vi "Listbox.vi"(0 "Items":i32(listbox), 5 "Selected Item":string, 7 "error in (no error)":errorcluster) -> (4 "error out":errorcluster)   [LabVIEW 2020]
doc: "This VI has a string control which moves over the row selected in the listbox."
panel:
  # "Select a row to get the string control \nover the selected row."
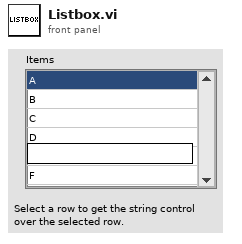
[diagram p1: front panel]
types:
  T1 = typedef "LVPositionTypeDef.ctl" = cluster{"Left":i32, "Top":i32}
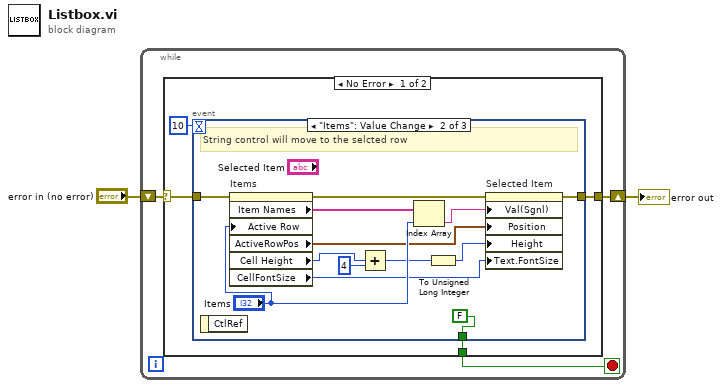
[diagram p0: block diagram]
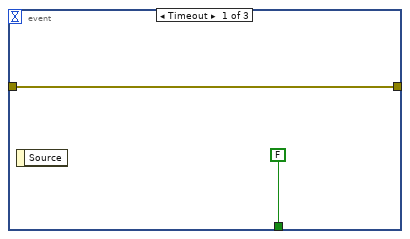
[diagram p2: hidden frame]
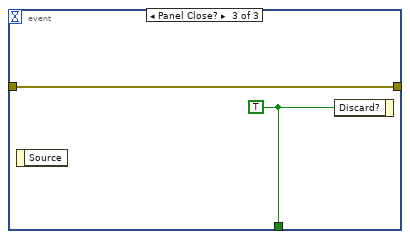
[diagram p3: hidden frame]
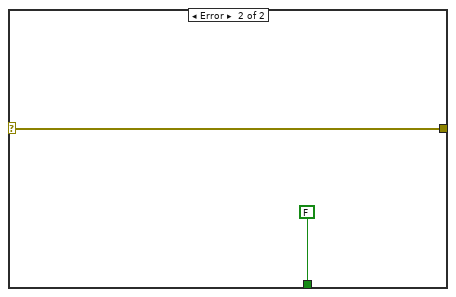
[diagram p4: hidden frame]
diagram:
  n1 = while {
    shift-right: [w5] -> w2
    shift-left: "error in (no error)" -> [w4]
    stop <- w3 stop-if-true
    n2 = case shown="No Error" w4 {
      selector: w4 -> [w8 w28]
      tunnel: [w9 w28] -> w5
      tunnel: [w6 FALSE ("Discard?")] -> w3
      frame No Error {
        n3 = event shown="[1] \"Items\": Value Change" {
          selector: _ -> [_ _ _]
          dyn-events: _ -> [_ _ _]
          timeout: 10 -> [_ _ _]
          tunnel: w8 -> [w11 w22 w25]
          tunnel: [w11 w21 w25] -> w9
          tunnel: [FALSE ("Discard?") FALSE ("Discard?") w26] -> w6
          event Timeout {
            n4 = event-data() -> ()  [unwired: 1 in, 1 out]
          }
          event "Items": Value Change {
            # "String control will move to the selcted row"
            n5 = event-data() -> ()  [unwired: 1 in, 1 out]
            n6 = property on="Items" class="LstBox (strict)"(error in=w22, "Active Row"="Items") -> (error out=w19:errorcluster, "Item Names"=w24:string[], "ActiveRowPos"=w17:T1, "Cell Height"=w13:i32, "CellFontSize"=w15:u32)  [unwired: 1 in, 1 out]
            n7 = Add(x=w13, y=4) -> (x+y=w14:i32)
            n8 = Index Array(array=w24, index="Items") -> (element=w23:string)
            n9 = To Unsigned Long Integer(number=w14) -> (unsigned 32bit integer=w16:u32)
            n10 = property on="Selected Item" class="Str"(error in=w19, "Val(Sgnl)"=w23, "Position"=w17, "Height"=w16, "Text.FontSize"=w15) -> (error out=w21:errorcluster)  [unwired: 1 in, 1 out]
          }
          event Panel Close? {
            w26 = TRUE ("Discard?")
            n11 = event-data() -> ()  [unwired: 1 in, 1 out]
            n12 = event-data("Discard?"=w26) -> ()  [unwired: 1 in, 1 out]
          }
        }
      }
      frame Error {
      }
    }
  }
  "error out" <- w2
